vi "GOMDBTS2048 spectral Get Spectrum Calibrated Wavelength.vi"(8 "error in (no error)":errorcluster, 11 "handle":i32) -> (0 "error out":errorcluster, 2 "function return":i32, 3 "spectrum":dbl[](array[numeric]))   [LabVIEW 2015, in "GOMDBTS2048.lvlib"]
doc: "GOBTS2048DLL int __stdcall GOMDBTS2048_spectralGetSpectrumCalibratedWavelength(int handle, double* spectrum);"
uses:
  GOMDBTS2048.lvlib
  runtime/GOMDBTS2048.dll
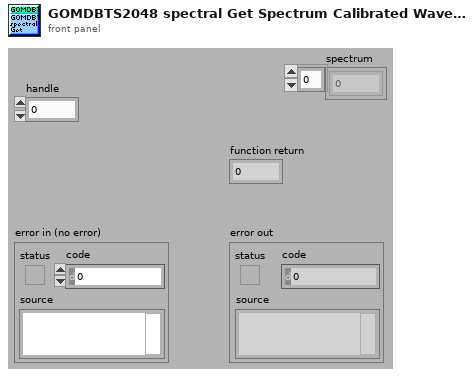
[diagram p1: front panel]
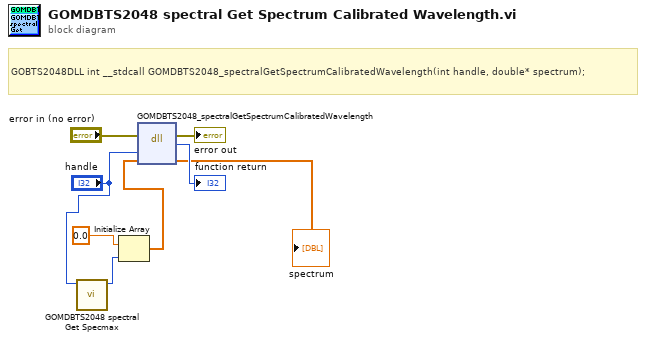
[diagram p0: block diagram]
diagram:
  # "GOBTS2048DLL int __stdcall GOMDBTS2048_spectralGetSpectrumCalibratedWavelength(int handle, double* spectrum);"
  n1 = call "GOMDBTS2048 spectral Get Specmax.vi"("handle"="handle") -> ("value"=w2:i32)  [unwired: 8 in, 2 out]
  n2 = Initialize Array(0.0 ("element"), w2) -> (w4:dbl[])
  n3 = dll-call lib="C:/Users/rkoch/Documents/GO_Library/runtime/GOMDBTS2048.*" fn="GOMDBTS2048_spectralGetSpectrumCalibratedWavelength"(error in="error in (no error)", "handle"="handle", "spectrum"=w4) -> (error out=→"error out":errorcluster, "return type"=→"function return":i32, "spectrum"=→"spectrum":dbl[])  [unwired: 3 in, 1 out]
